vi "Measurement_Timing.vi"(1 "Last reading time":dbl format="%#_13g") -> (0 "Last reading time out":dbl format="%#_13g")   [LabVIEW 2016]
uses:
  Instrument_Setup.vi
panel:
  in  "Time":dbl=0.5 format="%#_13g"
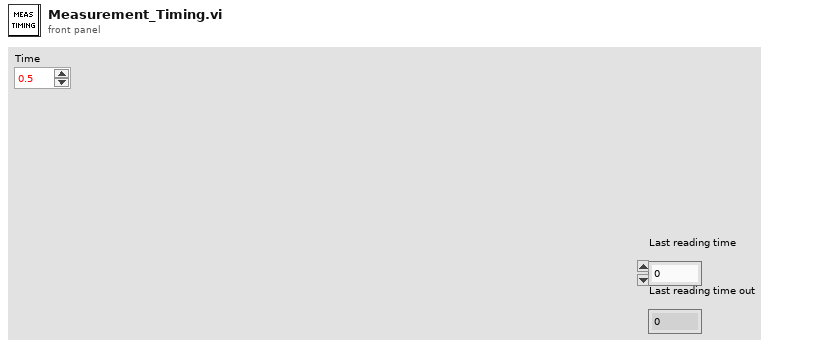
[diagram p1: front panel]
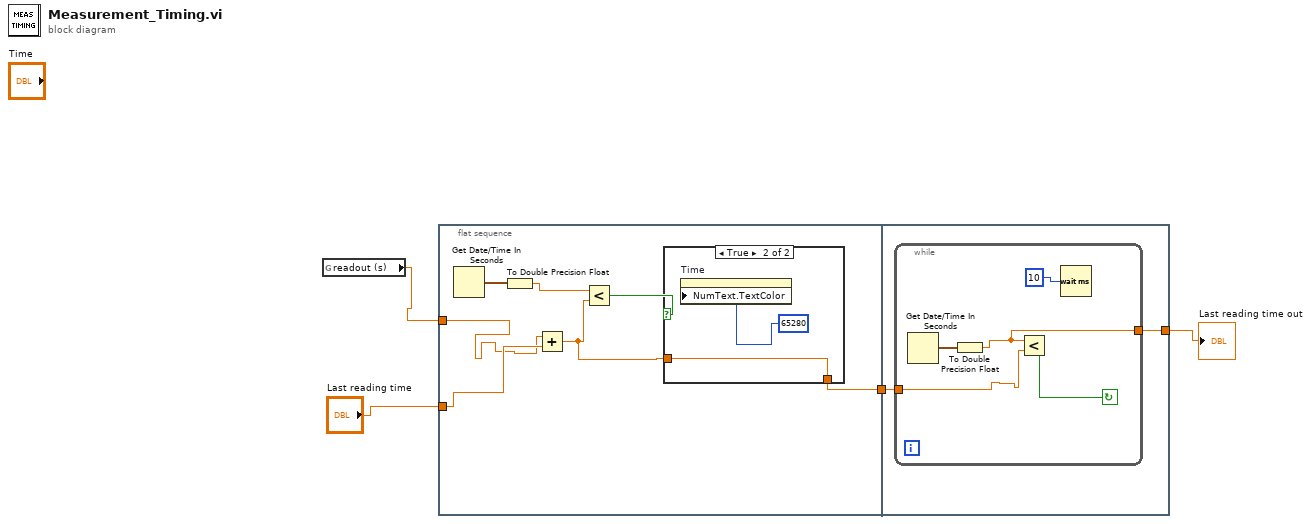
[diagram p0: block diagram]
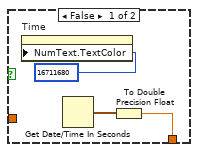
[diagram p2: hidden frame]
diagram:
  n1 = global read "Instrument_Setup.vi" "readout (s)"() -> (w1:dbl)
  n2 = flat-sequence {
    tunnel: "Last reading time" -> [w8]
    tunnel: [w6] -> w4
    tunnel: w1 -> [w5]
    tunnel: w4 -> [w18]
    tunnel: [w17] -> w2
    frame #0 {
      n3 = Get Date/Time In Seconds() -> (seconds since 1Jan1904=w11:timestamp)
      n4 = To Double Precision Float(number=w11) -> (double precision float=w10:dbl)
      n5 = Add(x=w5, y=w8) -> (x+y=w7:dbl)
      n6 = Less?(x=w10, y=w7) -> (x < y?=w9:bool)
      n7 = case shown="True" w9 {
        tunnel: w7 -> [_ w15]
        tunnel: [w12 w15] -> w6
        frame False {
          n8 = property on="Time" class="DigNum (strict)"("NumText.TextColor"=16711680) -> ()  [unwired: 2 in, 2 out]
          n9 = Get Date/Time In Seconds() -> (seconds since 1Jan1904=w13:timestamp)
          n10 = To Double Precision Float(number=w13) -> (double precision float=w12:dbl)
        }
        frame True {
          n11 = property on="Time" class="DigNum (strict)"("NumText.TextColor"=65280) -> ()  [unwired: 2 in, 2 out]
        }
      }
    }
    frame #1 {
      n12 = while {
        tunnel: w18 -> [w21]
        tunnel: [w20] -> w17
        stop <- w22 continue-if-true
        n13 = Get Date/Time In Seconds() -> (seconds since 1Jan1904=w23:timestamp)
        n14 = To Double Precision Float(number=w23) -> (double precision float=w20:dbl)
        n15 = Less?(x=w20, y=w21) -> (x < y?=w22:bool)
        n16 = Wait (ms)(milliseconds to wait=10) -> ()  [unwired: 1 out]
      }
    }
  }
  "Last reading time out" <- w2
